vi "SetBufferTimestampResolution.vi"(7 "SMU":T1, 8 "Error In":errorcluster, 9 "Resolution (sec)":dbl, 10 "Buffer":u8=1 min=1 max=2 step=1, 11 "Keithley 2602 In":refnum<visa-resource-name>) -> (0 "Error Out":errorcluster, 3 "Keithley 2602 Out":refnum<visa-resource-name>)   [LabVIEW 2012, in "Keithley-2602.lvlib"]
uses:
  Keithley-2602.lvlib
  Controls/SMU.ctl
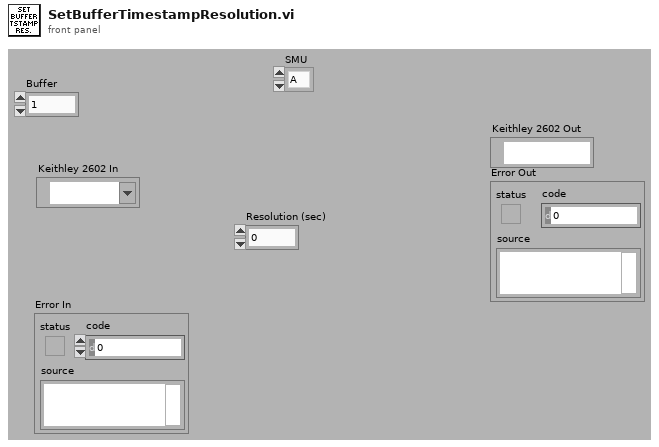
[diagram p1: front panel]
types:
  T1 = typedef "Keithley-2602.lvlib/SMU.ctl" = enum16{"A", "B"}
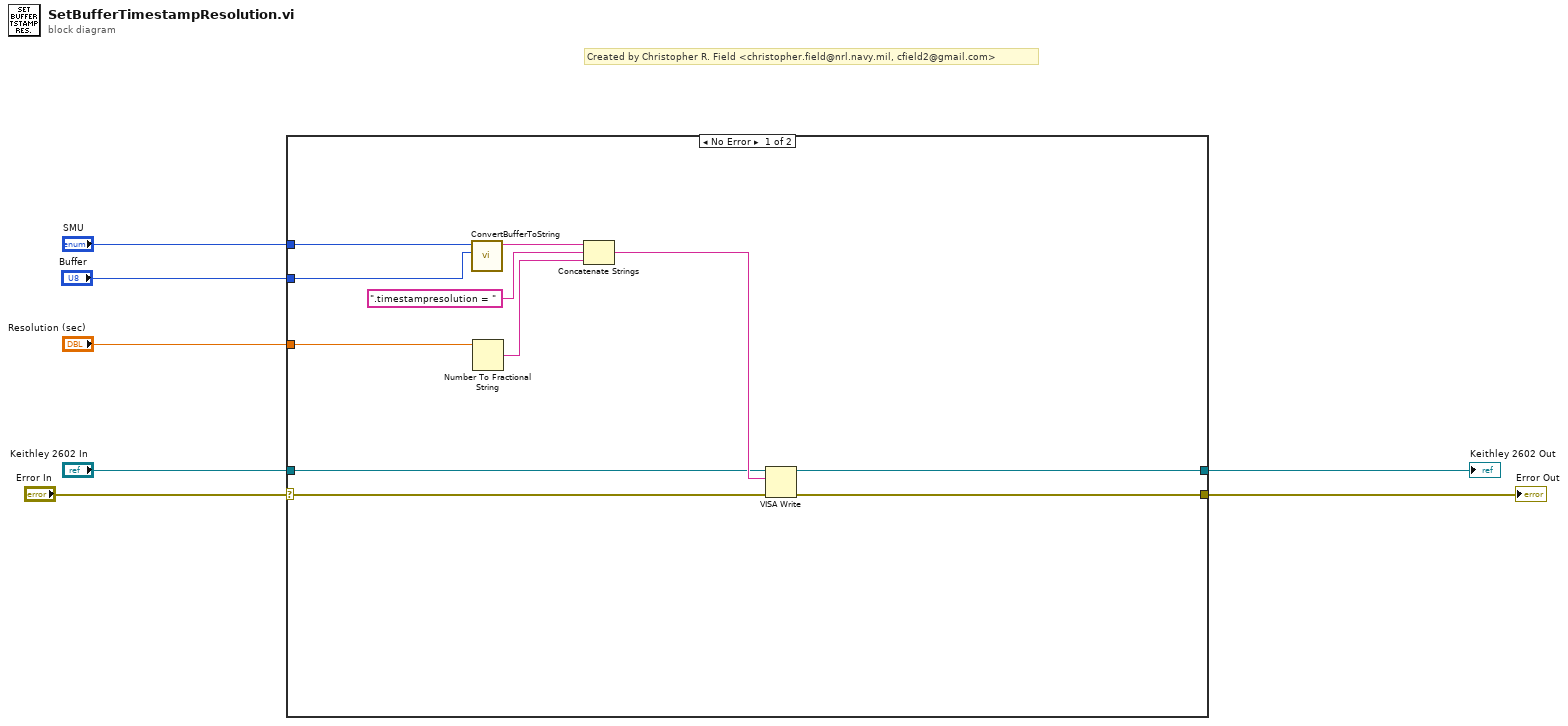
[diagram p0: block diagram]
diagram:
  # "Created by Christopher R. Field <christopher.field@nrl.navy.mil, cfield2@gmail.com>"
  n1 = case shown="No Error" "Error In" {
    selector: "Error In" -> [w8 w20]
    tunnel: "Keithley 2602 In" -> [w17 w19]
    tunnel: [w16 w19] -> w6
    tunnel: [w15 w20] -> w5
    tunnel: "Resolution (sec)" -> [w14 _]
    tunnel: "Buffer" -> [w10 _]
    tunnel: "SMU" -> [w9 _]
    frame No Error {
      n2 = call "ConvertBufferToString.vi"("Buffer"=w10, "SMU"=w9) -> ("Buffer"=w13:string)  [unwired: 9 in]
      n3 = Number To Fractional String(number=w14) -> (F-format string=w11:string)  [unwired: 3 in]
      n4 = Concatenate Strings(w13, ".timestampresolution = ", w11) -> (w18:string)
      n5 = VISA Write(VISA resource name=w17, write buffer=w18, error in (no error)=w8) -> (VISA resource name out=w16:refnum<visa-resource-name>, error out=w15:errorcluster)  [unwired: 1 out]
    }
    frame Error {
    }
  }
  "Keithley 2602 Out" <- w6
  "Error Out" <- w5
